vi "Draw Actor Core on Subpanel.vi"(8 "error in (no error)":errorcluster, 11 "Si UI in":refnum<class "Si UI.lvclass">) -> (0 "error out":errorcluster, 3 "Si UI out":refnum<class "Si UI.lvclass">)   [LabVIEW 2020, in "Si UI.lvlib" / "Si UI.lvclass"]
uses:
  Si UI.lvclass
  Si UI.lvclass/Si UI.ctl
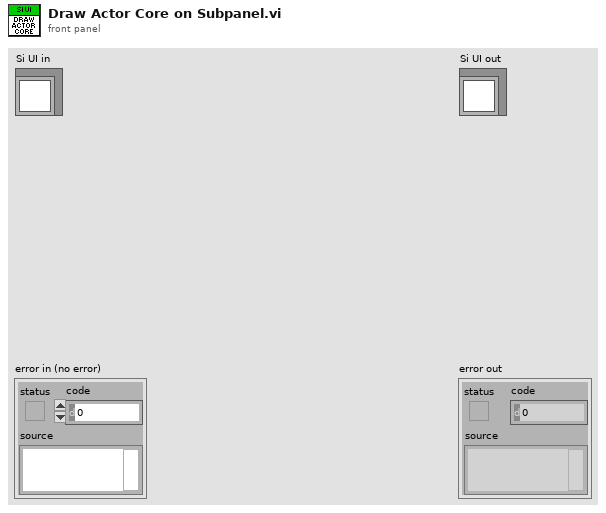
[diagram p1: front panel]
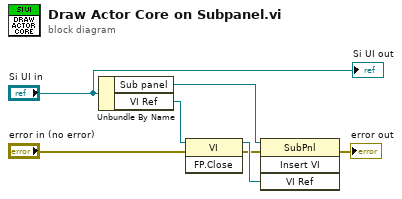
[diagram p0: block diagram]
diagram:
  n1 = Unbundle By Name("Si UI in") -> ("Sub panel"=w6:refnum<vi>, "VI Ref"=w4:refnum<vi>)
  n2 = invoke class="VI" method="FP.Close"(reference=w4, error in="error in (no error)") -> (reference out=w3:refnum<vi>, error out=w1:errorcluster)  [unwired: 1 in, 1 out]
  n3 = invoke class="SubPnl" method="Insert VI"(reference=w6, error in=w1, "VI Ref"=w3) -> (error out=→"error out":errorcluster)  [unwired: 1 in, 3 out]
  "Si UI out" <- "Si UI in"
